vi "Set Selected.vi"(6 "Get All Children?":bool=TRUE, 7 "Tri-State?":bool=TRUE, 8 "error in (no error)":errorcluster, 10 "Tag":string, 11 "Tree Reference":refnum<vi>) -> (0 "error out":errorcluster, 2 "Seted Tags":T1(array[cluster]), 3 "Tree Reference":refnum<vi>)   [LabVIEW 2023, in "DSLV_Tree.lvlib"]
uses:
  DSLV_Tree.lvlib
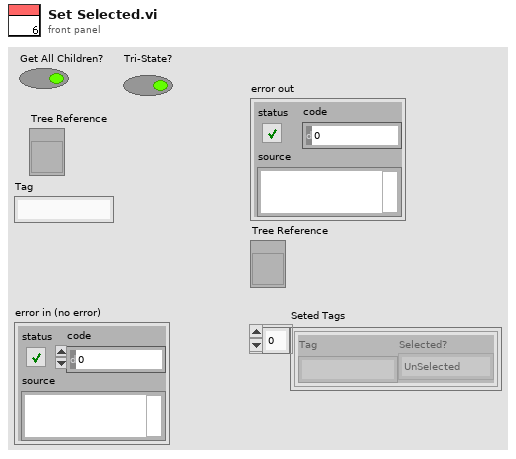
[diagram p1: front panel]
types:
  T1 = cluster{"Tag":string, "Selected?":enum16{"UnSelected", "Selected", "PartSelected"}}[]
  T2 = cluster{"Tag":string, "Selected?":enum16{"UnSelected", "Selected", "PartSelected"}}
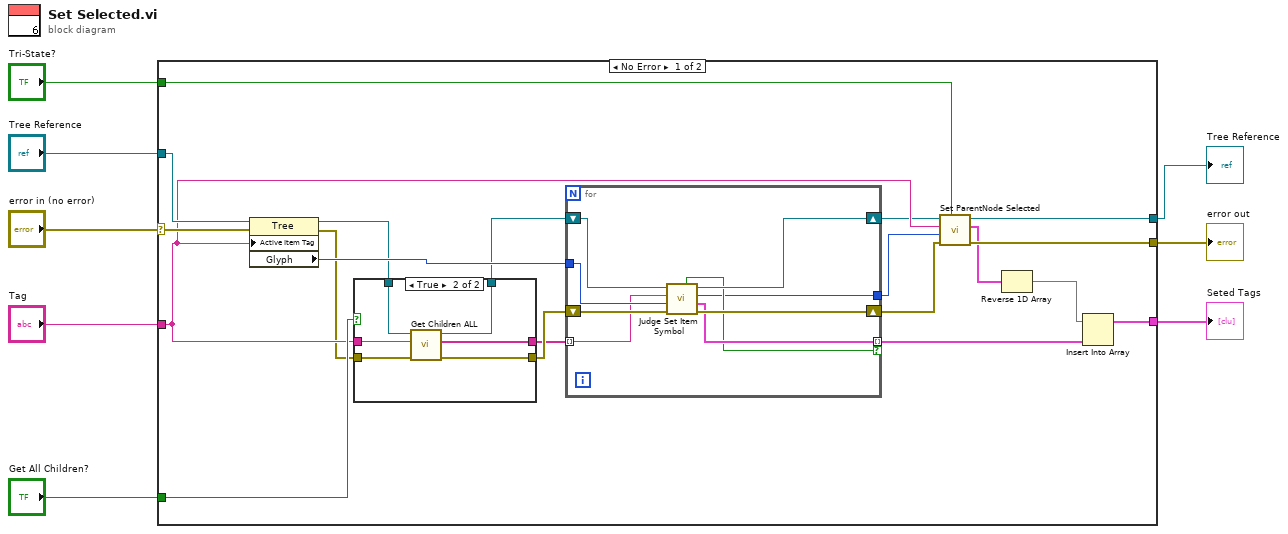
[diagram p0: block diagram]
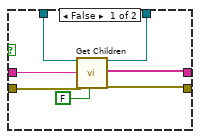
[diagram p2: hidden frame]
diagram:
  n1 = case shown="No Error" "error in (no error)" {
    selector: "error in (no error)" -> [w23 w51]
    tunnel: "Tree Reference" -> [w24 w52]
    tunnel: [w28 w51] -> w7
    tunnel: [w27 w52] -> w6
    tunnel: "Get All Children?" -> [w26 _]
    tunnel: [w25 _] -> w2
    tunnel: "Tag" -> [w22 _]
    tunnel: "Tri-State?" -> [w9 _]
    frame No Error {
      n2 = property on="Property Node" class="Tree"(reference=w24, error in=w23, "Active Item Tag"=w22) -> (reference out=w20:refnum<vi>, error out=w18:errorcluster, "Glyph"=w21:i32)
      n3 = case shown="True" w26 {
        tunnel: w20 -> [w34 w41]
        tunnel: [w33 w40] -> w19
        tunnel: w22 -> [w32 w39]
        tunnel: [w35 w38] -> w16
        tunnel: w18 -> [w31 w37]
        tunnel: [w29 w36] -> w17
        frame False {
          n4 = call "Get Children.vi"("Tree Reference In"=w34, "Parent Tag"=w32, "error in (no error)"=w31, "Use Current"=FALSE) -> ("Tree Reference Out"=w33:refnum<vi>, "Children Tags"=w35:string[], "error out"=w29:errorcluster)  [unwired: 13 in]
        }
        frame True {
          n5 = call "Get Children ALL.vi"("error in"=w37, "Parent Tag"=w39, "Tree Reference"=w41) -> ("error out"=w36:errorcluster, "Children Tags"=w38:string[], "Tree Reference"=w40:refnum<vi>)  [unwired: 6 in]
        }
      }
      n6 = for {
        tunnel: w21 -> [w50]
        shift-right: [w48] -> w14
        shift-left: w17 -> [w49]
        shift-right: [w47] -> w15
        shift-left: w19 -> [w46]
        tunnel: w16 -> [w42] mode=indexing
        tunnel: [w45] -> w12 mode=indexing if=w44
        tunnel: [w43] -> w13
        n7 = call "Judge Set Item Symbol.vi"("error in (no error)"=w49, "Symbol index"=w50, "Tag"=w42, "TreeControl in"=w46) -> ("error out"=w48:errorcluster, "Set out"=w45:T2, "New Symbol Index"=w43:i32, "TreeControl out"=w47:refnum<vi>, "Set?"=w44:bool)  [unwired: 3 in]
      }
      n8 = call "Set ParentNode Selected.vi"("Tri-State?"=w9, "error in (no error)"=w14, "Symbol Index"=w13, "Tag"=w22, "TreeControl in"=w15) -> ("error out"=w28:errorcluster, "Seted Tags"=w11:T1, "TreeControl out"=w27:refnum<vi>)  [unwired: 4 in]
      n9 = Reverse 1D Array(array=w11) -> (reversed array=w10:T1)
      n10 = Insert Into Array(array=w10, new element=w12) -> (w25:T1)  [unwired: 1 in]
    }
    frame Error {
    }
  }
  "error out" <- w7
  "Tree Reference" <- w6
  "Seted Tags" <- w2
